vi "IMAQ FPGA FIFO to Pixel Bus RGB32x1.vi"(6 "Ready For Output":bool=TRUE, 10 "Image Size":T3, 11 "Source Image FIFO":refnum<k21>) -> (0 "Output Valid":bool, 1 "Column":u32, 2 "Line":u32, 3 "Pixel Out":T1, 5 "Source FIFO Status":T2)   [LabVIEW 2015, in "NI_VDM_FPGA_Basics.lvlib"]
doc: "Reads image pixels out of the specified FIFO and returns a Pixel Bus cluster of the requested type. The Pixel Bus contains the pixel data from the FIFO along with some additional flags that indicate when the pixel data is valid, an end of a line has been reached, or an end of the image has been reached. The Pixel Bus is used to pass image data to all of the other VIs in the NI Vision Development Module for FPGA library. Only one of the DV, EOL, and EOI flags in the Pixel Bus cluster will assert on a given clock cycle. When the last pixel of an image is reached, the Pixel Bus will contain the pixel data and the DV flag will be TRUE and the EOL and EOI flags will be FALSE. The next clock cycle, the EOL flag will be TRUE and the DV and EOI flags will be FALSE. The following clock cycle, the EOI flag will be TRUE and the DV and EOL flags will be FALSE."
uses:
  <vilib>/visionFPGA/NI_VDM_FPGA_Basics.lvlib
  <vilib>/visionFPGA/Controls/IMAQ FPGA Image Size.ctl
  <vilib>/visionFPGA/Controls/IMAQ FPGA Source FIFO Status.ctl
  <vilib>/visionFPGA/Controls/IMAQ FPGA Pixel Bus u8x1.ctl
  <vilib>/rvi/DataTransferAndStorage/Container/Common/niFpgaContainerExecOnDevCompGetState.vi
  <vilib>/rvi/Emulation/niFpgaEmulationIsFPGAContextNoSignature.vi
  <vilib>/rvi/Emulation/niFpgaSctlEmulationGetInTimedLoop.vi
  <vilib>/rvi/errors/niFpgaSetErrorForExecOnDevCompSimple.vi
  <vilib>/rvi/eio/common/nirviEmuReportErrorAndStop.vi
  <vilib>/rvi/DataTransferAndStorage/Container/Common/niFpgaContainerGetUniqueNameForEmu.vi
  <vilib>/rvi/FIFO/Fifo_Resource/nirvififoEmulationSetSize.vi
  <vilib>/rvi/FIFO/Fifo_Resource/nirviFifoEmulationQueueMgr.vi
  <instcachedir>/0/nirviFifoEmulationQueueMgr_E5CAEC123FF24DC58D834DCA3CDAA9B5.lvgen/nirviFifoEmulationQueueMgr_E5CAEC123FF24DC58D834DCA3CDAA9B5_001.vi
  <vilib>/rvi/FIFO/Fifo_Resource/nirvififoEmulationDetermineInputValidOut.vi
  <vilib>/rvi/FIFO/Fifo_Resource/nirvififoEmulationCreateLock.vi
  <vilib>/rvi/Emulation/niFpgaProcessEmulError.vi
  <vilib>/rvi/FIFO/Fifo_Resource/nirvififoEmulationObtainLock.vi
  <vilib>/rvi/FIFO/Fifo_Resource/nirvififoEmulationReleaseLock.vi
  <vilib>/rvi/occurrence/nirviWaitOnOccurrenceBase.vi
  <vilib>/rvi/errors/nirviReportUnexpectedCaseInternalError.vi
  <vilib>/rvi/errors/nirviReportUnexpectedCaseInternalError (U32).vi
  <vilib>/Utility/error.llb/Clear Errors.vi
  <vilib>/rvi/interface/RandomDataEmulation/niFpgaRandomDataHandleErrors.vi
  <vilib>/rvi/DataTransferAndStorage/Container/XNode/niFpgaContainer.xnode
  <vilib>/rvi/FIFO/Fifo_Resource/niFpgaFifoEmulationRefIn.vi
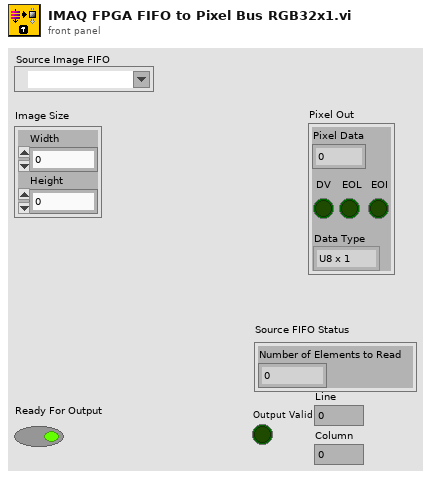
[diagram p1: front panel]
types:
  T1 = typedef "IMAQ FPGA Pixel Bus u8x1.ctl" = cluster{"Pixel Data":u8, "DV":bool, "EOL":bool, "EOI":bool, "Data Type":enum16{"U8 x 1"}}
  T2 = typedef "IMAQ FPGA Source FIFO Status.ctl" = cluster{"Number of Elements to Read":u32}
  T3 = typedef "IMAQ FPGA Image Size.ctl" = cluster{"Width":u32, "Height":u32}
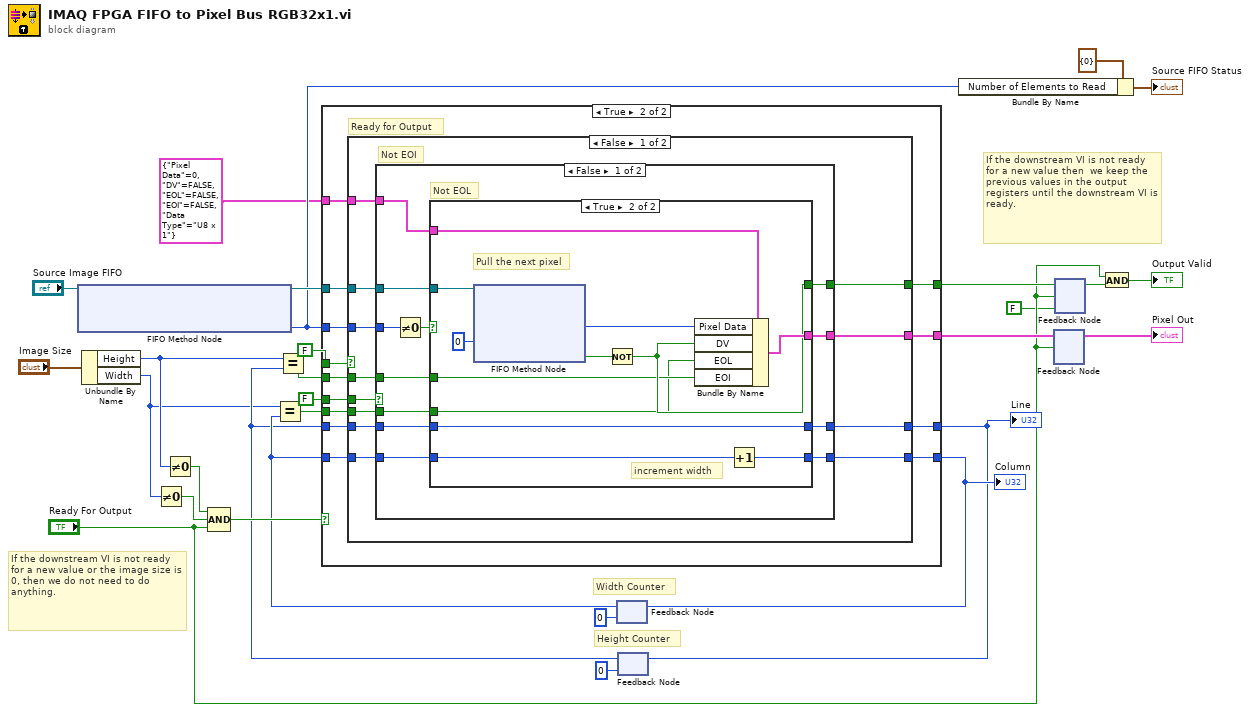
[diagram p0: block diagram]
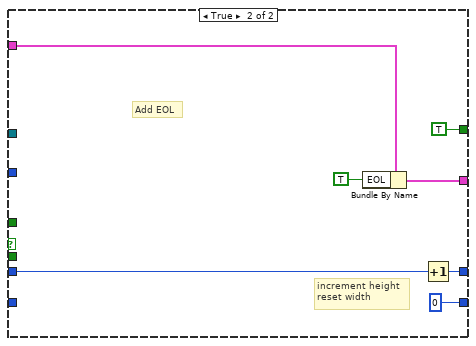
[diagram p4: hidden frame]
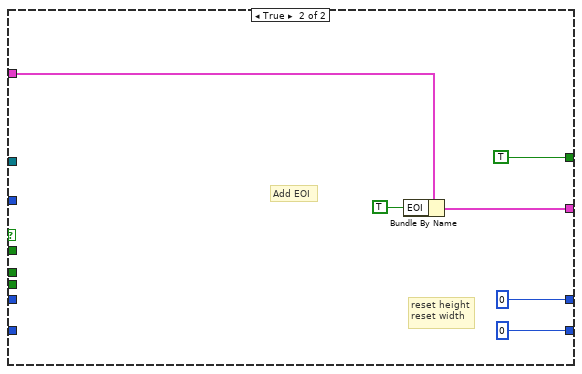
[diagram p5: hidden frame]
diagram:
  # "If the downstream VI is not ready for a new value or the image size is 0, then we do not need to do anything."
  # "If the downstream VI is not ready for a new value then  we keep the previous values in the output registers until the downstream VI is ready."
  # "Height Counter"
  # "Width Counter"
  n1 = xnode ("FIFO Method Node")("FIFO In"="Source Image FIFO") -> ("Number of Elements to Read"=w7:u32, "FIFO Out"=w23:refnum<k21>)
  n2 = Unbundle By Name("Image Size") -> ("Height"=w16:u32, "Width"=w15:u32)
  n3 = Not Equal To 0?(x=w15) -> (x != 0?=w21:bool)
  n4 = Not Equal To 0?(x=w16) -> (x != 0?=w20:bool)
  n5 = Compound Arithmetic op=AND(w20, w21, "Ready For Output") -> (w22:bool)
  n6 = feedback #1(u32 0 ("Image Width")) -> (w19:u32)
  n7 = Equal?(x=w15, y=w19) -> (x = y?=w3:bool)
  n8 = feedback #2(u32 0 ("Image Width")) -> (w18:u32)
  n9 = Equal?(x=w16, y=w18) -> (x = y?=w5:bool)
  n10 = case shown="True" w22 {
    tunnel: FALSE -> [_ w44]
    tunnel: T1 {"Pixel Data"=0, "DV"=FALSE, "EOL"=FALSE, "EOI"=FALSE, "Data Type"=enum."U8 x 1"} ("Red Plane Out") -> [_ w43]
    tunnel: FALSE -> [_ w42]
    tunnel: w7 -> [_ w41]
    tunnel: [_ w40] -> w28
    tunnel: [w30 w39] -> w26
    tunnel: w19 -> [w30 w38]
    tunnel: [w31 w37] -> w24
    tunnel: w18 -> [w31 w36]
    tunnel: [_ w35] -> w14
    tunnel: w23 -> [_ w34]
    tunnel: w5 -> [_ w33]
    tunnel: w3 -> [_ w32]
    frame False {
      # "Do nothing...\nDown stream VI is not ready for new data."
    }
    frame True {
      # "Ready for Output"
      n11 = case shown="False" w44 {
        tunnel: w42 -> [w56 _]
        tunnel: [w55 TRUE ("EOI")] -> w40
        tunnel: [w54 w91] -> w35
        tunnel: w36 -> [w53 _]
        tunnel: w38 -> [w52 _]
        tunnel: [w51 u16 0 ("Height Counter")] -> w37
        tunnel: [w50 u16 0 ("Width Counter")] -> w39
        tunnel: w41 -> [w49 _]
        tunnel: w43 -> [w48 w90]
        tunnel: w34 -> [w47 _]
        tunnel: w33 -> [w46 _]
        tunnel: w32 -> [w45 _]
        frame False {
          # "Not EOI"
          n12 = case shown="False" w56 {
            tunnel: [w66 w88] -> w54
            tunnel: [w65 TRUE ("EOI")] -> w55
            tunnel: w53 -> [w64 w86]
            tunnel: w52 -> [w63 _]
            tunnel: [w61 w84] -> w51
            tunnel: [w62 u16 0 ("Width Counter")] -> w50
            tunnel: w49 -> [w67 _]
            tunnel: w48 -> [w60 w83]
            tunnel: w47 -> [w59 _]
            tunnel: w46 -> [w58 _]
            tunnel: w45 -> [w57 _]
            frame False {
              # "Not EOL"
              n13 = Not Equal To 0?(x=w67) -> (x != 0?=w68:bool)
              n14 = case shown="True" w68 {
                tunnel: [_ w81] -> w66
                tunnel: [_ w74] -> w65
                tunnel: w64 -> [w69 w78]
                tunnel: w63 -> [w70 w80]
                tunnel: [w70 w79] -> w62
                tunnel: [w69 w78] -> w61
                tunnel: w60 -> [_ w76]
                tunnel: w59 -> [_ w75]
                tunnel: w58 -> [_ w73]
                tunnel: w57 -> [_ w72]
                frame False {
                  # "Do nothing...\nnot EOI, not EOL, \nand no DMA data available"
                }
                frame True {
                  # "increment width"
                  # "Pull the next pixel"
                  n15 = xnode ("FIFO Method Node")("Timeout"=0, "FIFO In"=w75) -> ("Element"=w71:u8, "Timed Out?"=w77:bool)  [unwired: 1 out]
                  n16 = Not(x=w77) -> (.not. x?=w74:bool)
                  n17 = Bundle By Name(cluster=w76, "Pixel Data"=w71, "DV"=w74, "EOL"=w72, "EOI"=w73) -> (w81:T1)
                  n18 = Increment(x=w80) -> (x+1=w79:u32)
                }
              }
            }
            frame True {
              # "increment height\nreset width"
              # "Add EOL"
              n19 = Bundle By Name(cluster=w83, "EOL"=TRUE) -> (w88:T1)
              n20 = Increment(x=w86) -> (x+1=w84:u32)
            }
          }
        }
        frame True {
          # "reset height\nreset width"
          # "Add EOI"
          n21 = Bundle By Name(cluster=w90, "EOI"=TRUE) -> (w91:T1)
        }
      }
    }
  }
  "Line" <- w24
  "Column" <- w26
  n22 = feedback-in #1(w26) -> ()
  n23 = feedback-in #2(w24) -> ()
  n24 = Bundle By Name(cluster=T2 {"Number of Elements to Read"=0} ("FIFO Status"), "Number of Elements to Read"=w7) -> (→"Source FIFO Status":T2)
  n25 = feedback-in #3(w14, "Ready For Output") -> ()
  n26 = feedback #3() -> (→"Pixel Out":T1)  [unwired: 1 in]
  n27 = feedback-in #4(w28, "Ready For Output") -> ()
  n28 = feedback #4(FALSE ("EOI")) -> (w12:bool)
  n29 = And(x="Ready For Output", y=w12) -> (x .and. y?=→"Output Valid":bool)
